vi "New Regex Filter.vi"   [LabVIEW 2018, in "GLog.lvlib" / "Regex.lvclass"]
doc: "Create a new Filter which matches log calls based on the contents of the Message field."
uses:
  Regex.lvclass
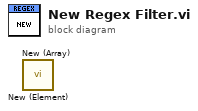
[diagram p0: block diagram]
diagram:
  n1 = call "New (Element).vi"() -> ()  [unwired: 10 in, 2 out]
  n2 = call "New (Array).vi"() -> ()  [unwired: 10 in, 2 out]
